vi "READ Config from XML file.vi"(8 "error in (no error)":errorcluster, 10 "Path":path, 11 "Default Op Config":T1={"Use Tool Cfg"=FALSE, "Use Tool Cal"=FALSE, "Fake Data?"=FALSE, "Mode"=-2, "Array Subset Length"=30, "nArrays to Read"=2, "Full Array Read Length"=500, "nSubarrays/Sensor"=0}) -> (0 "error out":errorcluster, 1 "Tool Op Config":T1={"Use Tool Cfg"=FALSE, "Use Tool Cal"=FALSE, "Fake Data?"=FALSE, "Mode"=-2, "Array Subset Length"=90, "nArrays to Read"=2, "Full Array Read Length"=512, "nSubarrays/Sensor"=0}, 2 "Found":bool, 5 "Cfg Cluster Version":string)   [LabVIEW 2015, in "Tool Module.lvlib"]
uses:
  Tool Module.lvlib
  Tool Config/_Tool Operation Config Cluster--typedef.ctl
  Tool Config/_Configuration Cluster_v1--typedef.ctl
  Tool Config/_Tool Block Cluster--typedef.ctl
  Tool Config/_Motor Block Cluster_v1--typedef.ctl
  Tool Config/_Verification Blk Cluster--typedef.ctl
  Tool Config/_Probe Block Cluster--typedef.ctl
  Tool Config/_ProbeConfigParams Cluster--typedef.ctl
  Tool Config/_Sensor Block Cluster--typedef.ctl
  Tool Config/_SensorConfigParams Cluster--typedef.ctl
  <vilib>/Utility/error.llb/Error Cluster From Error Code.vi
  <vilib>/Utility/xml.llb/Read From XML File(array).vi
  <vilib>/ErrorRing/Error Ring.xnode
  Tool Config/Tool Cfg.lvlib
panel:
  out "element":string
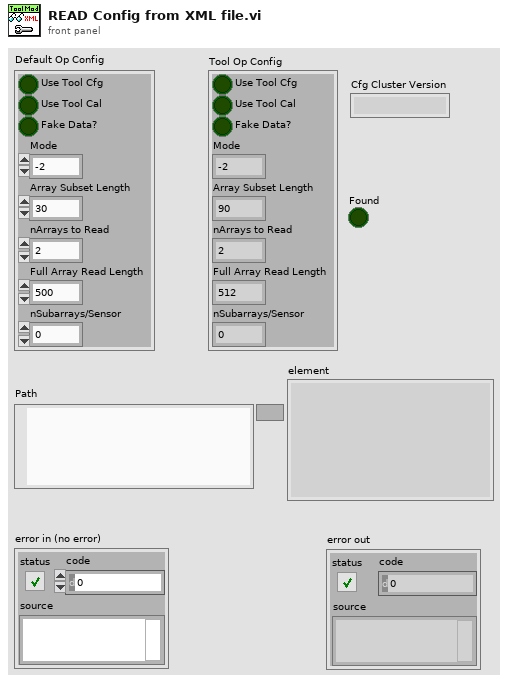
[diagram p1: front panel]
types:
  T1 = typedef "Tool Cfg.lvlib/_Tool Operation Config Cluster--typedef.ctl" = cluster{"Use Tool Cfg":bool, "Use Tool Cal":bool, "Fake Data?":bool, "Mode":i16, "Array Subset Length":i16, "nArrays to Read":i16, "Full Array Read Length":i16, "nSubarrays/Sensor":i16}
  T2 = typedef "Tool Cfg.lvlib/_Configuration Cluster_v1--typedef.ctl" = cluster{"Tool Type":u16, "Tool SN":u16, "Tool Block":T3, "Motor Block":T4, "Verification Block":T5, "Probe Block":T6}
  T3 = typedef "Tool Cfg.lvlib/_Tool Block Cluster--typedef.ctl" = cluster{"Encoder Size":u16, "Encoder Scale":u32, "Encoder Offset":i32, "MaxEncoder":i32, "MinEncoder":i32, "Start Delay":sgl}
  T4 = typedef "Tool Cfg.lvlib/_Motor Block Cluster_v1--typedef.ctl" = cluster{"MinMotor Speed":u16, "MaxMotor Speed":u16, "Homing Speed":u16, "Jog Speed":u16, "Inspect Speed":u16, "VBlk Speed":u16, "CleaningPos":i32, "Has Motor":bool, "Use Home Index":bool}
  T5 = typedef "Tool Cfg.lvlib/_Verification Blk Cluster--typedef.ctl" = cluster{"Angle":sgl, "FlankLength1":sgl, "FlankLength2":sgl, "Location":sgl, "Serial Number":u16}
  T6 = typedef "Tool Cfg.lvlib/_Probe Block Cluster--typedef.ctl" = cluster{"nProbes":u16, "Probe Param Array":T7[]}
  T7 = typedef "Tool Cfg.lvlib/_ProbeConfigParams Cluster--typedef.ctl" = cluster{"Name":string, "Laser Init Pwr":u16, "Laser Gain":u8, "Integ Count":u16, "Meas. Range":sgl, "Angle":sgl, "Probe Offset":sgl, "Sensor Block":T8}
  T8 = typedef "Tool Cfg.lvlib/_Sensor Block Cluster--typedef.ctl" = cluster{"nSensors":u16, "SensorCfgParams Array":T9[]}
  T9 = typedef "Tool Cfg.lvlib/_SensorConfigParams Cluster--typedef.ctl" = cluster{"Total Pixels":u16, "Positive  Peaks":bool, "CalibrCoefArray":dbl[], "Start Idx":u16, "End Idx":u16}
  T10 = typedef "Tool Cfg.lvlib/_Configuration Cluster_v2--typedef.ctl" = cluster{"Tool Type":u16, "Tool SN":u16, "Tool Block":T3, "Motor Block":T11, "Verification Block":T5, "Probe Block":T6}
  T11 = typedef "Tool Cfg.lvlib/_Motor Block Cluster_v2--typedef.ctl" = cluster{"MinMotor Speed":u16, "MaxMotor Speed":u16, "Homing Speed":u16, "Jog Speed":u16, "Inspect Speed":u16, "VBlk Speed":u16, "CleaningPos":i32, "Safe Zone":i32, "Has Motor":bool, "Use Home Index":bool}
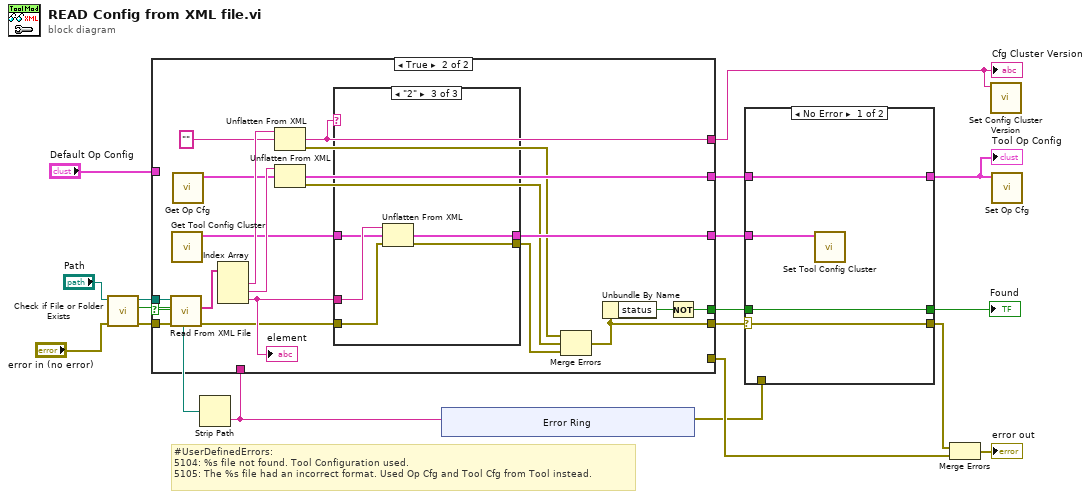
[diagram p0: block diagram]
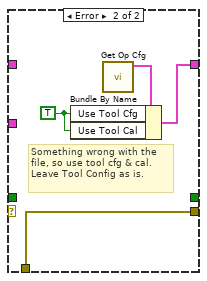
[diagram p2: hidden frame]
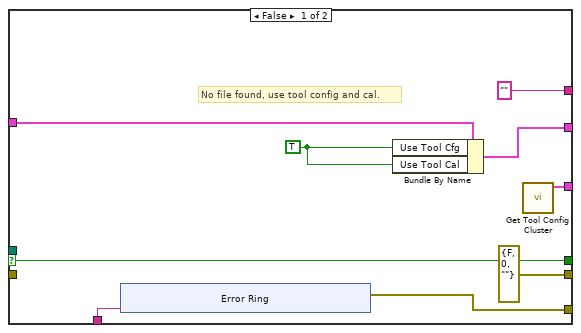
[diagram p3: hidden frame]
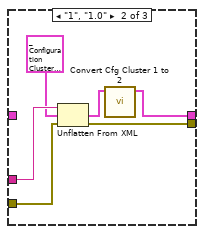
[diagram p5: hidden frame]
diagram:
  # "#UserDefinedErrors:\n5104: %s file not found. Tool Configuration used.\n5105: The %s file had an incorrect format. Used Op Cfg and Tool Cfg from Tool instead."
  n1 = call <vilib>:"Check if File or Folder Exists.vi"("error in (no error)"="error in (no error)", "path"="Path") -> ("error out"=w5:errorcluster, "file or folder exists?"=w6:bool, "dup path"=w13:path)  [unwired: 7 in]
  n2 = Strip Path(path=w13) -> (name=w14:string)  [unwired: 1 out]
  n3 = case shown="True" w6 {
    selector: w6 -> [w27 _]
    tunnel: [errorcluster {"status"=FALSE, "code"=0, "source"=""} ("error IO") w50] -> w8
    tunnel: w13 -> [_ w52]
    tunnel: w5 -> [_ w51]
    tunnel: [w27 w48] -> w4
    tunnel: "Default Op Config" -> [w25 _]
    tunnel: [w24 w47] -> w9
    tunnel: [w19 w46] -> w10
    tunnel: ["" w35] -> w1
    tunnel: w14 -> [w22 _]
    tunnel: [w20 _] -> w16
    frame False {
      w26 = TRUE ("Use Tool Cfg")
      # "No file found, use tool config and cal."
      n4 = xnode "Error Ring"("parameter 0"=w22) -> ("error out"=w20:errorcluster)
      n5 = Bundle By Name(cluster=w25, "Use Tool Cfg"=w26, "Use Tool Cal"=w26) -> (w24:T1)
      n6 = call "Get Tool Config Cluster.vi"() -> ("Tool Config Cluster"=w19:T10)  [unwired: 11 in]
    }
    frame True {
      n7 = call-poly <vilib>:"Read From XML File.vi"("error in (no error)"=w51, "XML File Path"=w52) -> ("error out"=w38:errorcluster, "XML Elements"=w53:string[])  [unwired: 7 in, 1 out]
      n8 = call "Get Tool Config Cluster.vi"() -> ("Tool Config Cluster"=w39:T10)  [unwired: 11 in]
      n9 = call "Get Op Cfg.vi"() -> ("Tool Operation Config"=w36:T1)  [unwired: 11 in]
      n10 = Index Array(array=w53) -> (element #1=w42:string, element #2=w44:string, element #3=w45:string)  [unwired: 3 in]
      "element" <- w45
      n11 = Unflatten From XML(xml string=w42, type="") -> (value=w35:string, error out=w43:errorcluster)  [unwired: 1 in]
      n12 = Unflatten From XML(xml string=w44, type=w36) -> (value=w47:T1, error out=w41:errorcluster)  [unwired: 1 in]
      n13 = case shown="\"2\"" w35 {
        tunnel: [w55 w56 w66] -> w46
        tunnel: w45 -> [_ w61 w65]
        tunnel: [w54 w58 w64] -> w40
        tunnel: w39 -> [w55 _ w63]
        tunnel: w38 -> [w54 w59 w62]
        frame Default {
        }
        frame "1", "1.0" {
          n14 = Unflatten From XML(xml string=w61, type=T2 {"Tool Type"=0, "Tool SN"=0, "Tool Block"={"Encoder Size"=0, "Encoder Scale"=0, "Encoder Offset"=0, "MaxEncoder"=0, "MinEncoder"=0, "Start Delay"=0.0}, "Motor Block"={"MinMotor Speed"=0, "MaxMotor Speed"=0, "Homing Speed"=90, "Jog Speed"=90, "Inspect Speed"=90, "VBlk Speed"=90, "CleaningPos"=0, "Has Motor"=FALSE, "Use Home Index"=FALSE}, "Verification Block"={"Angle"=90.0, "FlankLength1"=0.0, "FlankLength2"=0.0, "Location"=0.0, "Serial Number"=0}, "Probe Block"={"nProbes"=0, "Probe Param Array"=[]}} ("_Tool Config Cluster_v1--typedef"), error in (no error)=w59) -> (value=w57:T2, error out=w58:errorcluster)
          n15 = call "Convert Cfg Cluster 1 to 2.vi"("Tool Config Cluster_v1"=w57) -> ("Tool Config Cluster_v2"=w56:T10)  [unwired: 10 in]
        }
        frame "2" {
          n16 = Unflatten From XML(xml string=w65, type=w63, error in (no error)=w62) -> (value=w66:T10, error out=w64:errorcluster)
        }
      }
      n17 = Merge Errors(w43, w41, w40) -> (w50:errorcluster)
      n18 = Unbundle By Name(w50) -> ("status"=w49:bool)
      n19 = Not(x=w49) -> (.not. x?=w48:bool)
    }
  }
  "Cfg Cluster Version" <- w1
  n20 = xnode "Error Ring"("parameter 0"=w14) -> ("error out"=w15:errorcluster)
  n21 = case shown="No Error" w8 {
    selector: w8 -> [w69 _]
    tunnel: [w70 w74] -> w2
    tunnel: w9 -> [w70 _]
    tunnel: w10 -> [w67 _]
    tunnel: w15 -> [_ w72]
    tunnel: [w69 w72] -> w17
    tunnel: w4 -> [w68 _]
    tunnel: [w68 _] -> w3
    frame No Error {
      n22 = call "Set Tool Config Cluster.vi"("Tool Config Cluster"=w67) -> ()  [unwired: 11 in]
    }
    frame Error {
      w73 = TRUE ("Use Tool Cfg")
      # "Something wrong with the\nfile, so use tool cfg & cal.\nLeave Tool Config as is."
      n23 = call "Get Op Cfg.vi"() -> ("Tool Operation Config"=w71:T1)  [unwired: 11 in]
      n24 = Bundle By Name(cluster=w71, "Use Tool Cfg"=w73, "Use Tool Cal"=w73) -> (w74:T1)
    }
  }
  "Found" <- w3
  "Tool Op Config" <- w2
  n25 = Merge Errors(w17, w16) -> (→"error out":errorcluster)
  n26 = call "Set Config Cluster Version.vi"("Config Cluster Version"=w1) -> ()  [unwired: 11 in]
  n27 = call "Set Op Cfg.vi"("Tool Operation Config"=w2) -> ()  [unwired: 11 in]
